vi "Read Address.vi"(7 "Number of Addresses to read (1)":u8=1, 8 "error in (no error)":errorcluster, 9 "Address number (0)":u8 max=49, 10 "Motor ID (0)":u8, 11 "Dynamixel Motor VISA in":refnum<class "Dynamixel Motor VISA.lvclass">) -> (0 "error out":errorcluster, 1 "Motor Error Status":T1, 2 "Data Read":u8[](array[numeric]), 3 "Dynamixel Motor VISA out":refnum<class "Dynamixel Motor VISA.lvclass">)   [LabVIEW 2016, in "Dynamixel Motor VISA.lvclass"]
doc: "Reads an arbitrary number of consecutive addresses from a motor's register. This is a Low-Level VI that is used by other VIs."
uses:
  <instrlib>/Dynamixel Motor/HAIOL/VISA/Dynamixel Motor VISA.lvclass
  <instrlib>/Dynamixel Motor/Public/Motor Operation/Low Level/Alarm Setting.ctl
  <instrlib>/Dynamixel Motor/HAIOL/VISA/Dynamixel Motor VISA.lvclass/Dynamixel Motor VISA.ctl
  <instrlib>/Dynamixel Motor/Dynamixel Motor.lvlib
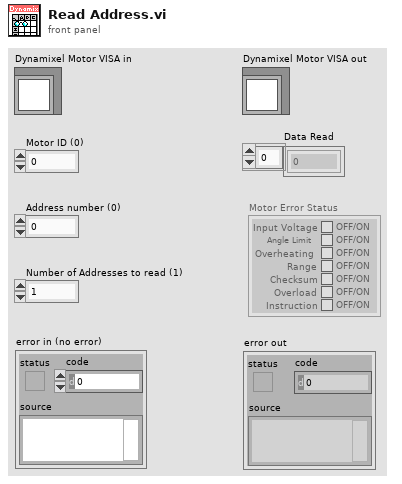
[diagram p1: front panel]
types:
  T1 = typedef "Dynamixel Motor.lvlib/Alarm Setting.ctl" = cluster{"Input Voltage":bool, "Angle Limit":bool, "Overheating ":bool, "Range":bool, "Checksum":bool, "Overload":bool, "Instruction":bool}
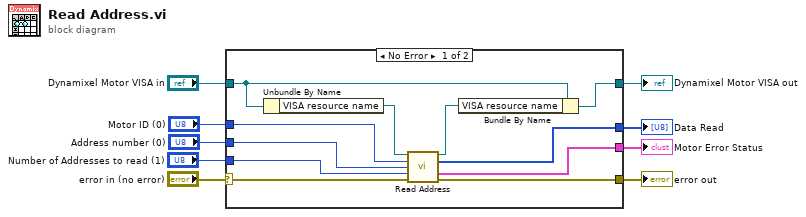
[diagram p0: block diagram]
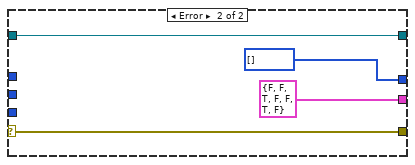
[diagram p2: hidden frame]
diagram:
  n1 = case shown="No Error" "error in (no error)" {
    selector: "error in (no error)" -> [w20 w21]
    tunnel: "Dynamixel Motor VISA in" -> [w11 w24]
    tunnel: "Motor ID (0)" -> [w18 _]
    tunnel: "Address number (0)" -> [w17 _]
    tunnel: "Number of Addresses to read (1)" -> [w16 _]
    tunnel: [w15 w21] -> w4
    tunnel: [w14 u8[] [] ("Data Read")] -> w3
    tunnel: [w13 T1 {"Input Voltage"=FALSE, "Angle Limit"=FALSE, "Overheating "=TRUE, "Range"=FALSE, "Checksum"=FALSE, "Overload"=TRUE, "Instruction"=FALSE} ("Motor Error Status")] -> w2
    tunnel: [w10 w24] -> w1
    frame No Error {
      n2 = Unbundle By Name(w11) -> ("VISA resource name"=w19:refnum<visa-resource-name>)
      n3 = call <instrlib>:"Read Address.vi"("VISA resource name"=w19, "Motor ID (0)"=w18, "Address number (0)"=w17, "Number of Addresses to read (1)"=w16, "Error in (no error)"=w20) -> ("VISA resource name Out"=w12:refnum<visa-resource-name>, "Data Read"=w14:u8[], "Motor Error Status"=w13:T1, "error out"=w15:errorcluster)  [unwired: 7 in]
      n4 = Bundle By Name(cluster=w11, "VISA resource name"=w12) -> (w10:refnum<class "Dynamixel Motor VISA.lvclass">)
    }
    frame Error {
    }
  }
  "error out" <- w4
  "Dynamixel Motor VISA out" <- w1
  "Motor Error Status" <- w2
  "Data Read" <- w3
